vi "SetParameter.vi"(7 "Camera Parameter":T1, 8 "error in (no error)":errorcluster, 10 "Value":i32, 11 "Stream in":refnum<class "Stream.lvclass">) -> (0 "error out":errorcluster, 1 "Set Value":i32, 3 "Stream":refnum<class "Stream.lvclass">)   [LabVIEW 2020, in "capture.lvlib" / "Stream.lvclass"]
doc: "SetParameter."
uses:
  Stream.lvclass
  Camera Parameters.ctl
  Stream.lvclass/Stream.ctl
  common/common.lvlib
  common/bin/gartoolkit_32-1.dll
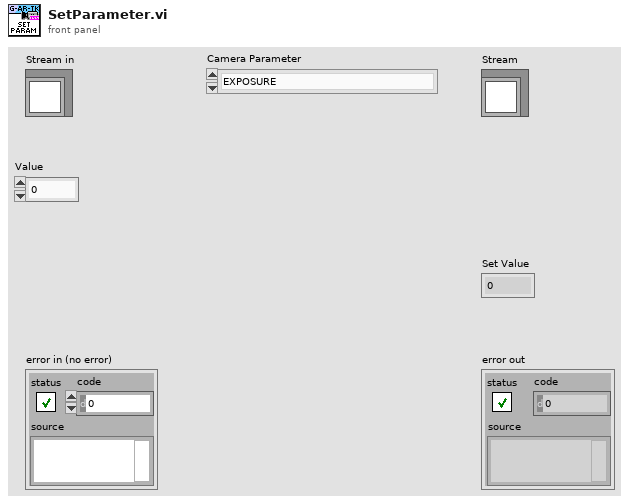
[diagram p1: front panel]
types:
  T1 = typedef "capture.lvlib/Stream.lvclass/Camera Parameters.ctl" = enum8{"EXPOSURE", "FOCUS", "ZOOM", "GAIN", "WHITE_BALANCE_TEMPERATURE", "BRIGHTNESS", "CONTRAST", "SATURATION", "GAMMA", "HUE", "SHARPNESS", "BACKLIGHT_COMPENSATION", "POWER_LINE_FREQUENCY"}
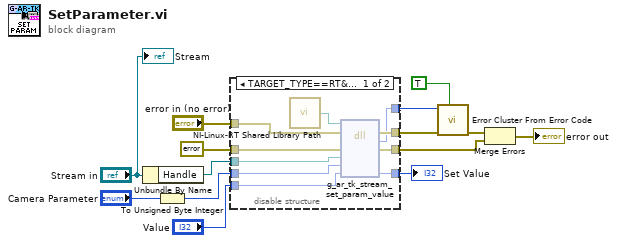
[diagram p0: block diagram]
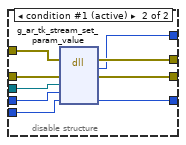
[diagram p2: hidden frame]
diagram:
  n1 = Unbundle By Name("Stream in") -> ("Handle"=w8:refnum<data-value>)
  n2 = To Unsigned Byte Integer(number="Camera Parameter") -> (unsigned 8bit integer=w7:u8)
  n3 = disable-structure shown="TARGET_TYPE==RT&&OS==Linux" {
    disable-tunnel: "error in (no error)" -> [w23 w33]
    disable-tunnel: errorcluster {"status"=FALSE, "code"=0, "source"=""} ("error constant") -> [w22 w32]
    disable-tunnel: w8 -> [w21 w31]
    disable-tunnel: w7 -> [w20 w30]
    disable-tunnel: "Value" -> [w19 w29]
    disable-tunnel: [w18 w28] -> w5
    disable-tunnel: [w17 w27] -> w4
    disable-tunnel: [w16 w26] -> w3
    disable-tunnel: [w15 w25] -> w2
    frame condition #0 {
      n4 = call "NI-Linux-RT Shared Library Path.vi"() -> ("Path"=w24:path)
      n5 = dll-call lib="?" fn="g_ar_tk_stream_set_param_value" ("g_ar_toolkit.*.*:g_ar_tk_stream_capture_next")(path in=w24, error in=w23, "error_cluster"=w22, "EDVR_strm"=w21, "parameter"=w20, "value"=w19) -> (error out=w18:errorcluster, "MgErr"=w17:i32, "error_cluster"=w16:errorcluster, "value"=w15:i32)  [unwired: 3 in, 1 out]
    }
    frame condition #1 (active) {
      n6 = dll-call lib="C:/serenial/lib/g-augmented-reality-toolkit/LabVIEW/common/bin/gartoolkit_*-1.*" fn="g_ar_tk_stream_set_param_value" ("g_ar_toolkit.*.*:g_ar_tk_stream_capture_next")(error in=w33, "error_cluster"=w32, "EDVR_strm"=w31, "parameter"=w30, "value"=w29) -> (error out=w28:errorcluster, "MgErr"=w27:i32, "error_cluster"=w26:errorcluster, "value"=w25:i32)  [unwired: 4 in, 1 out]
    }
  }
  "Set Value" <- w2
  n7 = call <vilib>:"Error Cluster From Error Code.vi"("show call chain? (False)"=TRUE, "error in (no error)"=w5, "error code (0)"=w4) -> ("error out"=w12:errorcluster)  [unwired: 6 in]
  n8 = Merge Errors(w12, w3) -> (→"error out":errorcluster)
  "Stream" <- "Stream in"
